vi "move_and_wait.vi"(8 "Error IN":errorcluster, 10 "MOVE TO POSITION":i32, 11 "VISA Resource IN":refnum<visa-resource-name>="COM1") -> (0 "Error OUT":errorcluster, 2 "CURRENT POSITION":i32, 3 "Visa Resource OUT":refnum<visa-resource-name>)   [LabVIEW 2013]
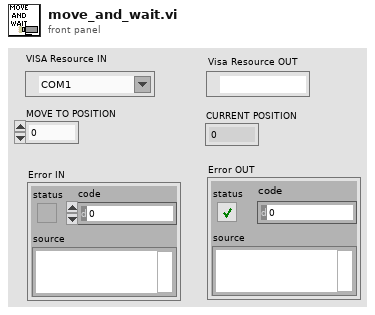
[diagram p1: front panel]
types:
  T1 = enum16{"Move to Home", "Set Positions", "Set Actuator Mode", "OTHER", "Set Direction", "CW Move", "CCW Move"}
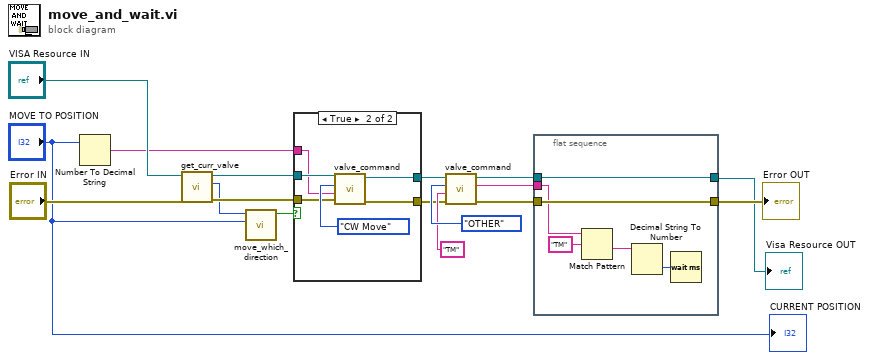
[diagram p0: block diagram]
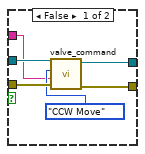
[diagram p2: hidden frame]
diagram:
  n1 = Number To Decimal String(number="MOVE TO POSITION") -> (decimal integer string=w4:string)  [unwired: 1 in]
  n2 = call "get_curr_valve.vi"("error in (no error)"="Error IN", "VALVE PORT IN"="VISA Resource IN") -> ("error out"=w6:errorcluster, "Current Valve"=w3:i32, "VALVE PORT OUT"=w5:refnum<visa-resource-name>)  [unwired: 7 in]
  n3 = call "move_which_direction.vi"("MOVE TO POSITION"="MOVE TO POSITION", "Current Valve"=w3) -> ("Move Clockwise?"=w1:bool)  [unwired: 9 in]
  n4 = case shown="True" w1 {
    tunnel: [w20 w28] -> w15
    tunnel: [w22 w27] -> w14
    tunnel: w6 -> [w21 w26]
    tunnel: w5 -> [w23 w25]
    tunnel: w4 -> [w18 w24]
    frame False {
      n5 = call "valve_command.vi"("Error IN"=w21, "Command option"=w18, "COMMANDS"=T1."CCW Move", "VALVE PORT IN"=w23) -> ("Error OUT"=w20:errorcluster, "VALVE PORT OUT"=w22:refnum<visa-resource-name>)  [unwired: 5 in, 1 out]
    }
    frame True {
      n6 = call "valve_command.vi"("Error IN"=w26, "Command option"=w24, "COMMANDS"=T1."CW Move", "VALVE PORT IN"=w25) -> ("Error OUT"=w28:errorcluster, "VALVE PORT OUT"=w27:refnum<visa-resource-name>)  [unwired: 5 in, 1 out]
    }
  }
  n7 = call "valve_command.vi"("Error IN"=w15, "Command option"="TM", "COMMANDS"=T1."OTHER", "VALVE PORT IN"=w14) -> ("Error OUT"=w12:errorcluster, "read buffer"=w13:string, "VALVE PORT OUT"=w10:refnum<visa-resource-name>)  [unwired: 5 in]
  n8 = flat-sequence {
    tunnel: w13 -> [w32]
    tunnel: w12 -> [w34]
    tunnel: [w34] -> w11
    tunnel: w10 -> [w33]
    tunnel: [w33] -> w9
    frame #0 {
      n9 = Match Pattern(string=w32, regular expression="TM") -> (after substring=w30:string)  [unwired: 4 out]
      n10 = Decimal String To Number(string=w30) -> (number=w35:i32)  [unwired: 2 in, 1 out]
      n11 = Wait (ms)(milliseconds to wait=w35) -> ()  [unwired: 1 out]
    }
  }
  "Error OUT" <- w11
  "Visa Resource OUT" <- w9
  "CURRENT POSITION" <- "MOVE TO POSITION"
